vi "FA_ConvertToTDC.vi"(8 "Error In":errorcluster, 11 "Config":T1) -> (0 "Error Out":errorcluster, 3 "TDC":T3)   [LabVIEW 2014, in "FA_TDC.lvlib"]
doc: "Converts from a general config to a TDC typedef"
uses:
  FA_TDC.lvlib
  FA_TDC.ctl
  FA_NativeTypes API/source/VI Source/FA_Config.ctl
  FA_LocalStore API/source/VI Source/FA_LSSpecialTypes.ctl
  FA_LocalStore API/source/VI Source/FA_LocalStore.lvlib
  FA_NativeTypes API/source/VI Source/FA_NativeTypes.lvlib
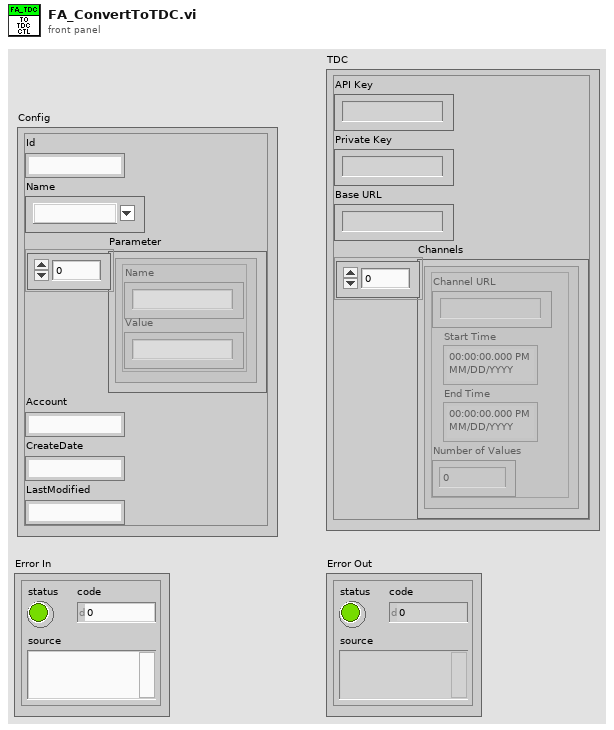
[diagram p1: front panel]
types:
  T1 = typedef "FA_NativeTypes.lvlib/FA_Config.ctl" = cluster{"Id":string, "Name":T2, "Parameter":cluster{"Name":string, "Value":string}[], "Account":string, "CreateDate":string, "LastModified":string}
  T2 = typedef "FA_LocalStore.lvlib/FA_LSSpecialTypes.ctl" = string
  T3 = typedef "FA_TDC.lvlib/FA_TDC.ctl" = cluster{"API Key":string, "Private Key":string, "Base URL":string, "Channels":cluster{"Channel URL":string, "Start Time":timestamp, "End Time":timestamp, "Number of Values":i32}[]}
  T4 = cluster{"Channel URL":string, "Start Time":timestamp, "End Time":timestamp, "Number of Values":i32}[]
  T5 = cluster{"Channel URL":string, "Start Time":timestamp, "End Time":timestamp, "Number of Values":i32}
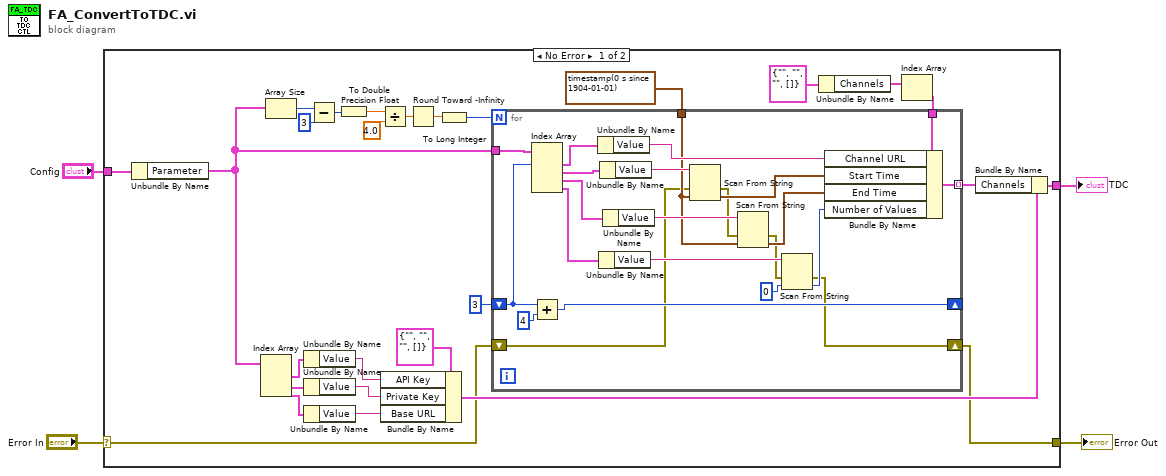
[diagram p0: block diagram]
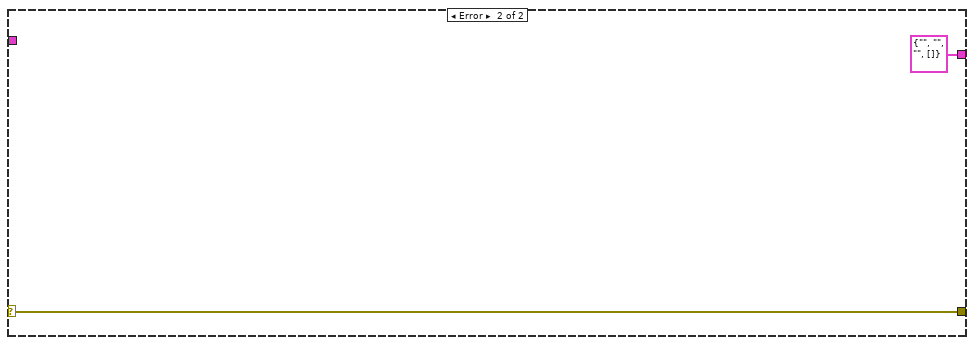
[diagram p2: hidden frame]
diagram:
  n1 = case shown="No Error" "Error In" {
    selector: "Error In" -> [w6 w55]
    tunnel: "Config" -> [w31 _]
    tunnel: [w11 T3 {"API Key"="", "Private Key"="", "Base URL"="", "Channels"=[]} ("TDC")] -> w2
    tunnel: [w5 w55] -> w1
    frame No Error {
      n2 = Unbundle By Name(w31) -> ("Parameter"=w20:cluster{"Name":string, "Value":string}[])
      n3 = Index Array(array=w20) -> (element #1=w26:cluster{"Name":string, "Value":string}, element #2=w25:cluster{"Name":string, "Value":string}, element #3=w24:cluster{"Name":string, "Value":string})  [unwired: 3 in]
      n4 = Array Size(array=w20) -> (size(s)=w30:i32)
      n5 = Unbundle By Name(w26) -> ("Value"=w23:string)
      n6 = Unbundle By Name(w25) -> ("Value"=w22:string)
      n7 = Unbundle By Name(w24) -> ("Value"=w21:string)
      n8 = Subtract(x=w30, y=3) -> (x-y=w28:i32)
      n9 = To Double Precision Float(number=w28) -> (double precision float=w9:dbl)
      n10 = Divide(x=w9, y=4.0) -> (x/y=w27:dbl)
      n11 = Bundle By Name(cluster=T3 {"API Key"="", "Private Key"="", "Base URL"="", "Channels"=[]} ("TDC"), "API Key"=w23, "Private Key"=w22, "Base URL"=w21) -> (w13:T3)
      n12 = Round Toward -Infinity(1:w27) -> (0:w19:dbl)
      n13 = To Long Integer(number=w19) -> (32bit integer=w18:i32)
      n14 = Unbundle By Name(T3 {"API Key"="", "Private Key"="", "Base URL"="", "Channels"=[]} ("TDC")) -> ("Channels"=w16:T4)
      n15 = Index Array(array=w16) -> (element=w15:T5)  [unwired: 1 in]
      n16 = for {
        N: w18 -> [_]
        tunnel: w20 -> [w52]
        tunnel: w15 -> [w49]
        tunnel: [w42] -> w12 mode=indexing
        tunnel: timestamp(0 s since 1904-01-01) ("default value 1") -> [w41]
        shift-right: [w36] -> _
        shift-left: 3 ("index") -> [w38]
        shift-right: [w32] -> w5
        shift-left: w6 -> [w35]
        n17 = Index Array(array=w52, index #1=w38) -> (element #1=w54:cluster{"Name":string, "Value":string}, element #2=w53:cluster{"Name":string, "Value":string}, element #3=w51:cluster{"Name":string, "Value":string}, element #4=w50:cluster{"Name":string, "Value":string})  [unwired: 3 in]
        n18 = Add(x=w38, y=4) -> (x+y=w36:i32)
        n19 = Unbundle By Name(w54) -> ("Value"=w48:string)
        n20 = Unbundle By Name(w50) -> ("Value"=w47:string)
        n21 = Unbundle By Name(w53) -> ("Value"=w45:string)
        n22 = Unbundle By Name(w51) -> ("Value"=w46:string)
        n23 = Scan From String(input string=w45, error in=w35, default 1=w41) -> (error out=w34:errorcluster, output 1=w44:timestamp)  [unwired: 2 in, 2 out]
        n24 = Scan From String(input string=w46, error in=w34, default 1=w41) -> (error out=w33:errorcluster, output 1=w40:timestamp)  [unwired: 2 in, 2 out]
        n25 = Scan From String(input string=w47, error in=w33, default 1=0 ("default value 1")) -> (error out=w32:errorcluster, output 1=w43:i32)  [unwired: 2 in, 2 out]
        n26 = Bundle By Name(cluster=w49, "Channel URL"=w48, "Start Time"=w44, "End Time"=w40, "Number of Values"=w43) -> (w42:T5)
      }
      n27 = Bundle By Name(cluster=w13, "Channels"=w12) -> (w11:T3)
    }
    frame Error {
    }
  }
  "TDC" <- w2
  "Error Out" <- w1
